vi "Comparator.vi"(0 "VISA resource name":refnum<visa-resource-name>, 1 "Mode (0: Absolute)":u32(ring) items=["Absolute", "Percent Tolerance", "Sequence"], 2 "Auxiliary Bin (F: Off)":bool, 3 "Swap (F: Off)":bool, 4 "Bin Sequence (0.1,0.2,0.3,0.4,0.5)":string="0.1,0.2,0.3,0.4,0.5", 5 "error in (no error)":errorcluster, 6 "Nominal Value (0.0)":dbl min=-9.9e+37 max=9.9e+37 step=1.0 format="%.4f", 7 "2nd Low Limit (0.0)":dbl min=-9.9e+37 max=9.9e+37 step=1.0 format="%.4f", 8 "Bin Number (0.0)":i16 min=0 max=9 step=1, 9 "2nd High Limit (0.0)":dbl min=-9.9e+37 max=9.9e+37 step=1.0 format="%.4f", 10 "Bin Low Limit (0.0)":dbl min=-9.9e+37 max=9.9e+37 step=1.0 format="%.4f", 12 "Bin High Limit (0.0)":dbl min=-9.9e+37 max=9.9e+37 step=1.0 format="%.4f") -> (14 "VISA resource name out":refnum<visa-resource-name>, 19 "error out":errorcluster)   [LabVIEW 2015, in "Agilent 428X Series.lvlib"]
doc: "The Comparator sets the comparator functions, including its limit mode and limits values."
uses:
  <instrlib>/Agilent 428X Series/Agilent 428X Series.lvlib
panel:
  # "On\nOff"
  # "On\nOff"
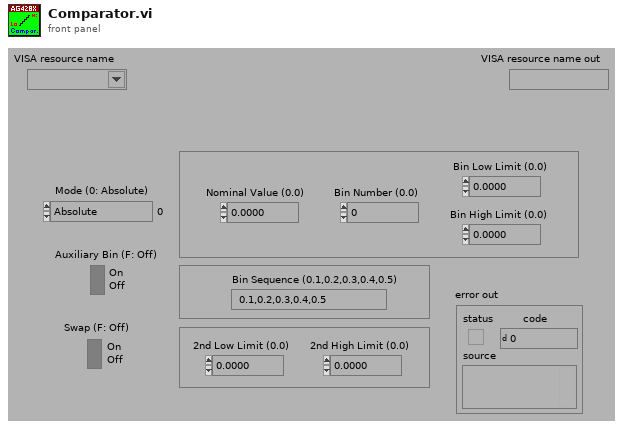
[diagram p1: front panel]
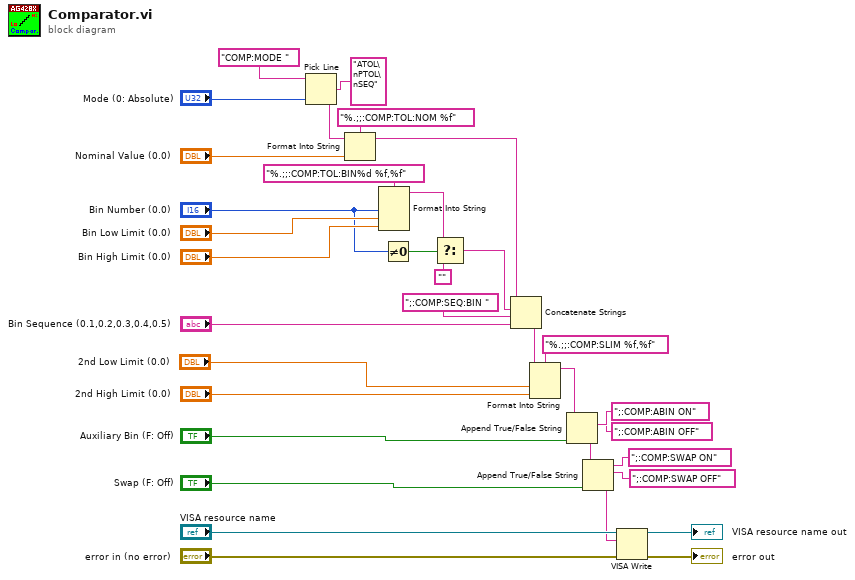
[diagram p0: block diagram]
diagram:
  n1 = Pick Line(string ("")="COMP:MODE ", multi-line string="ATOL\nPTOL\nSEQ", line index="Mode (0: Absolute)") -> (output string=w30:string)
  n2 = Format Into String(format string="%.;;:COMP:TOL:NOM %f", initial string=w30, "Nominal Value (0.0)") -> (resulting string=w1:string)  [unwired: 1 in, 1 out]
  n3 = Format Into String(format string="%.;;:COMP:TOL:BIN%d %f,%f", "Bin Number (0.0)", "Bin Low Limit (0.0)", "Bin High Limit (0.0)") -> (resulting string=w2:string)  [unwired: 2 in, 1 out]
  n4 = Not Equal To 0?(x="Bin Number (0.0)") -> (x != 0?=w24:bool)
  n5 = Select(t=w2, s=w24, f="") -> (s? t:f=w3:string)
  n6 = Concatenate Strings(w1, w3, ";:COMP:SEQ:BIN " ("Bin Sequence"), "Bin Sequence (0.1,0.2,0.3,0.4,0.5)") -> (w20:string)
  n7 = Format Into String(format string="%.;;:COMP:SLIM %f,%f", initial string=w20, "2nd Low Limit (0.0)", "2nd High Limit (0.0)") -> (resulting string=w12:string)  [unwired: 1 in, 1 out]
  n8 = Append True/False String(1:"Auxiliary Bin (F: Off)", 2:";:COMP:ABIN OFF", 3:";:COMP:ABIN ON", 4:w12) -> (0:w11:string)
  n9 = Append True/False String(1:"Swap (F: Off)", 2:";:COMP:SWAP OFF", 3:";:COMP:SWAP ON", 4:w11) -> (0:w4:string)
  n10 = VISA Write(VISA resource name="VISA resource name", write buffer=w4, error in (no error)="error in (no error)") -> (VISA resource name out=→"VISA resource name out":refnum<visa-resource-name>, error out=→"error out":errorcluster)  [unwired: 1 out]
